vi "listen_stop.vi"() -> ()   [LabVIEW 2019]
uses:
  global_str.vi
panel:
  out "源端口":u16
  out "源地址":u32
  out "接收数据":string
  out "错误输出 2":errorcluster={"status"=TRUE, "code"=1, "source"="listen_stop.vi中的关闭UDP"} caption="读取错误输出"
  out "错误输出":errorcluster={"status"=TRUE, "code"=54, "source"="listen_stop.vi中的打开UDP"} caption="监听错误输出"
  in  "监听地址":string="192.168.8.144"
  in  "监听端口":u16=4097
  in  "停止":bool
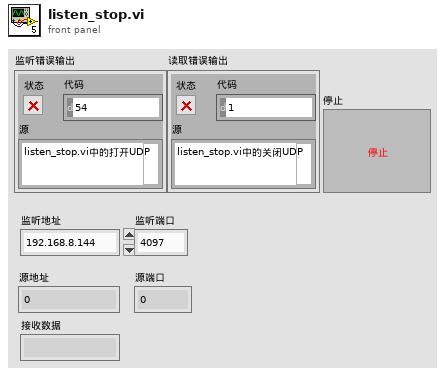
[diagram p1: front panel]
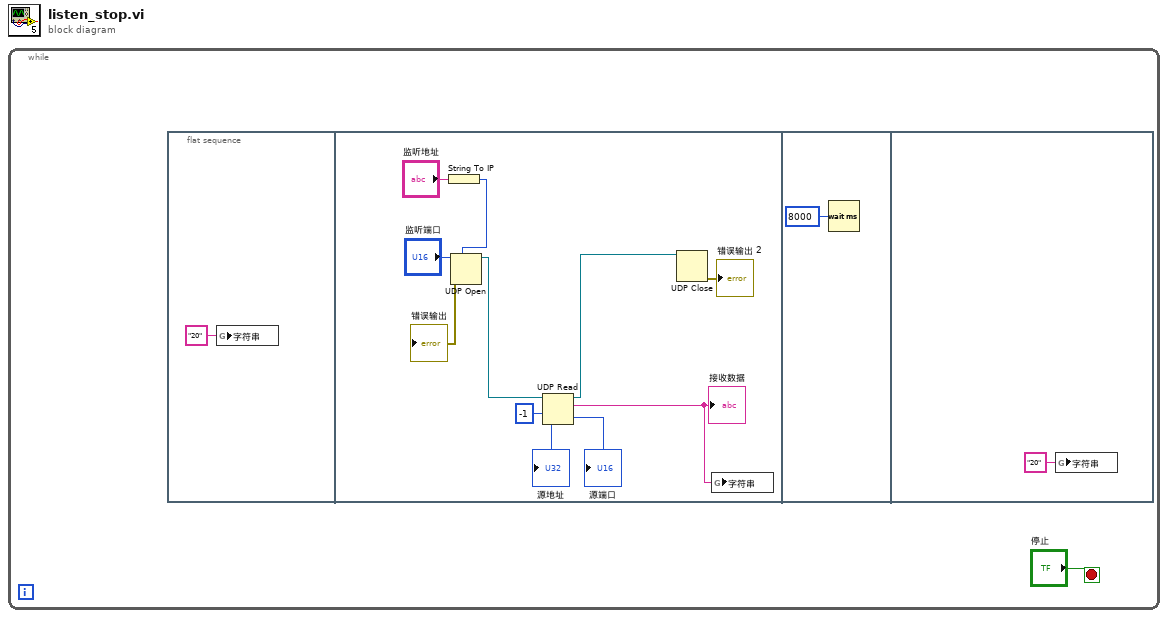
[diagram p0: block diagram]
diagram:
  n1 = while {
    stop <- "停止" stop-if-true
    n2 = flat-sequence {
      frame #0 {
        n3 = global write "global_str.vi" "字符串"("20" ("字符串")) -> ()
      }
      frame #1 {
        n4 = String To IP(1:"监听地址") -> (0:w4:u32)
        n5 = UDP Open(7:w4, 11:"监听端口") -> (port=w8:refnum<k16>, 0:→"错误输出":errorcluster)  [unwired: 3 in, 1 out]
        n6 = UDP Read(connection ID=w8, timeout ms (25000)=-1 ("超时毫秒(25000)")) -> (data out=w13:string, 3:w9:refnum<k16>, 4:→"源端口":u16, 6:→"源地址":u32)  [unwired: 2 in, 1 out]
        "接收数据" <- w13
        n7 = UDP Close(connection ID=w9) -> (error out=→"错误输出 2":errorcluster)  [unwired: 1 in, 1 out]
        n8 = global write "global_str.vi" "字符串"(w13) -> ()
      }
      frame #2 {
        n9 = Wait (ms)(milliseconds to wait=u32 8000 ("等待时间（毫秒）")) -> ()  [unwired: 1 out]
      }
      frame #3 {
        n10 = global write "global_str.vi" "字符串"("20" ("字符串")) -> ()
      }
    }
  }
